vi "Zaber A Series Joystick Configurator.vi"() -> ()   [LabVIEW 2015]
doc: "This VI is a helper for reading and changing the axis and button settings for an X-JOY3 joystick. It can also serve as an example for creating custom joystick initialization routines.\n\n<b>Note this tool only works with Zaber X-series joysticks such as the X-JOY3.</b>"
uses:
  Zaber A Series.lvlib
panel:
  out "Joystick Not \nDetected":bool
  out "Connected":bool
  in  "Joystick Device Number":string="1"
  in  "Disconnect":bool
  in  "VISA resource name":refnum<visa-resource-name>="COM1"
  in  "Connect":bool
  in  "Quit":bool
  in  "Tab Control":enum32{"Axes", "Buttons"}(tab)
  in  "Axis Tab":enum32{"Page 2"}(tab)
  in  "Joystick Axis":u32(ring)=1 items=["Left-Right"=1, "Forward-Back"=2, "Twist"=3]
  in  "Update Axis":bool
  in  "Target Axis Number":i32=1
  in  "Target Device Number":i32=2
  in  "Target Axis Type":u16(ring) items=["Axis", "Lockstep Group", "Virtual Axis"]
  in  "Maximum Speed":i32=100000
  in  "Speed Profile (0: No Change)":u16(ring) items=["No Change", "Linear", "Squared", "Cubed"]
  in  "Axis Direction (0: No Change)":u16(ring) items=["No Change", "Default Direction", "Inverted"]
  in  "Button Tab":enum32{"Page 2"}(tab)
  in  "Update Button":bool
  in  "Joystick Button Number":i32=1 min=1
  in  "Button Event":i32(ring)=1 items=["Pressed"=1, "Released"=2, "Held"=3, "Released After Hold"=4]
  in  "Command List":string[](array[string])
  # "(c) 2017 Zaber Technologies.  ALL RIGHTS RESERVED."
  # "This example allows you to view and edit the configuration of a Zaber ASCII-capable input device such as the X-JOY3.\n\nEnter the serial port and device number of the joystick at upper left and then press the Connect button.\n \nUse the controls in the Axes and Buttons tabs to view and change the settings on the joystick."
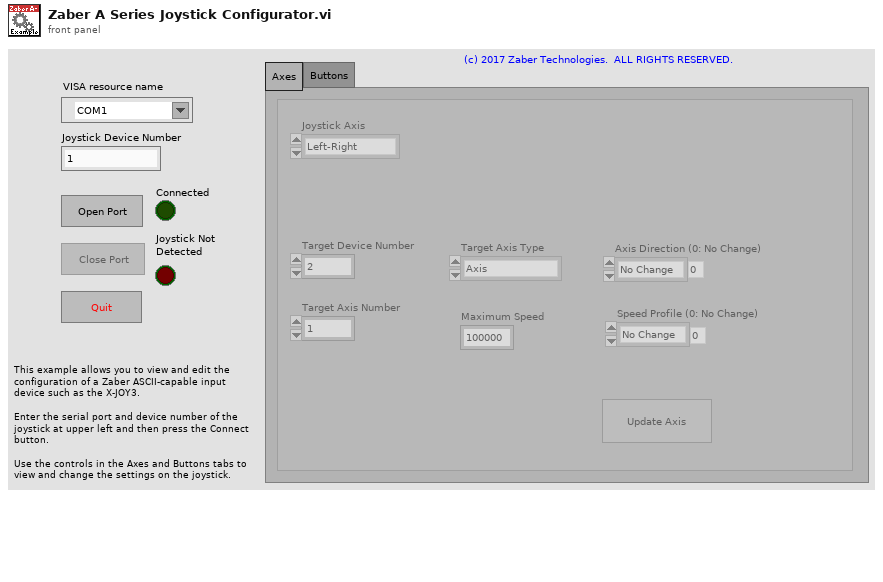
[diagram p1: front panel]
types:
  T1 = enum8{"Enabled", "Disabled", "Disabled and Grayed Out"}
  T2 = cluster{"Device":string, "Axis":string, "Reply Flag":string, "Status":string, "Warning Flags":string, "Data":string}
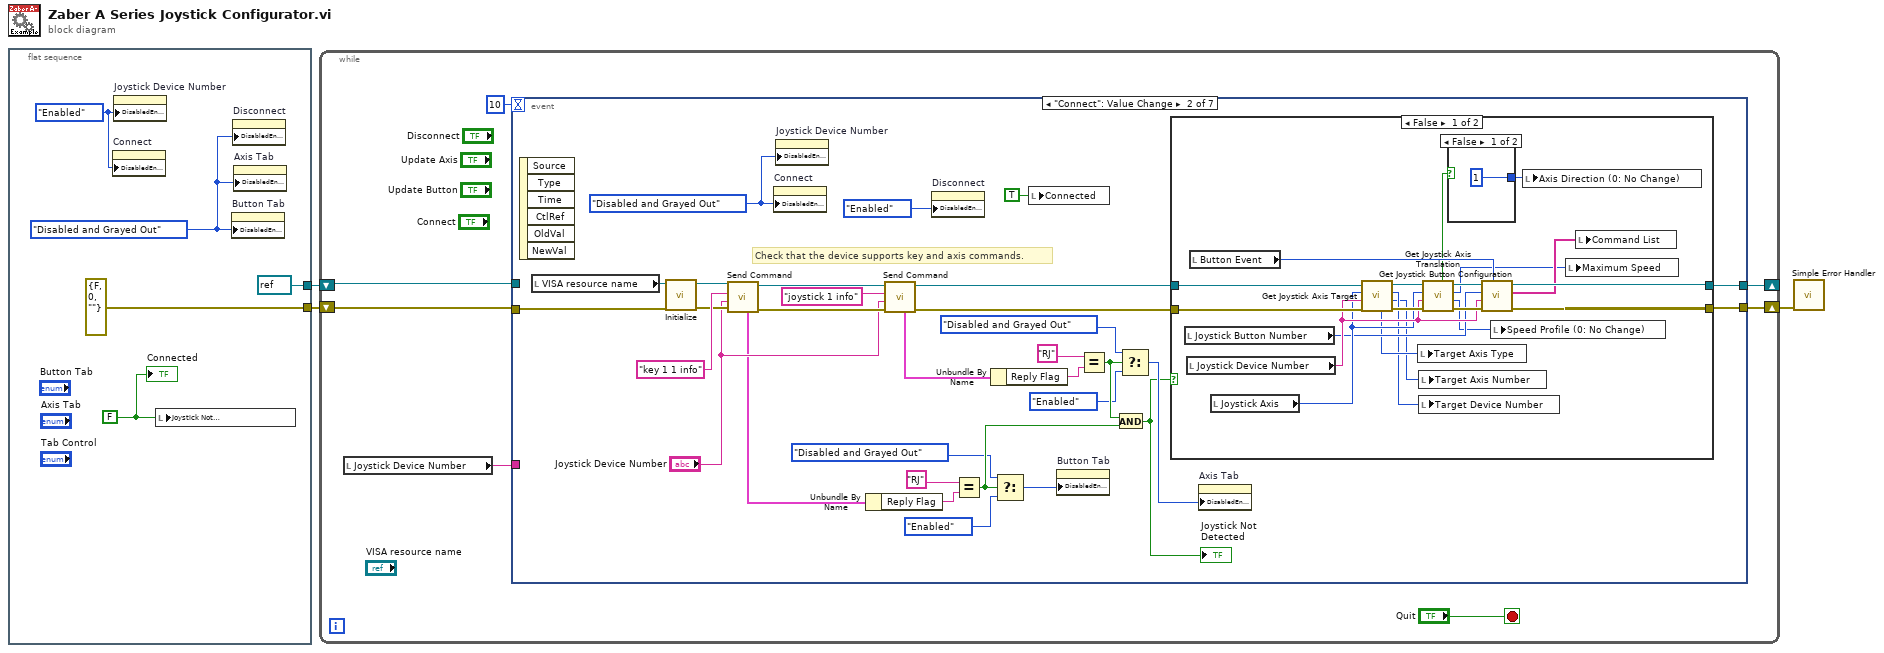
[diagram p0: block diagram]
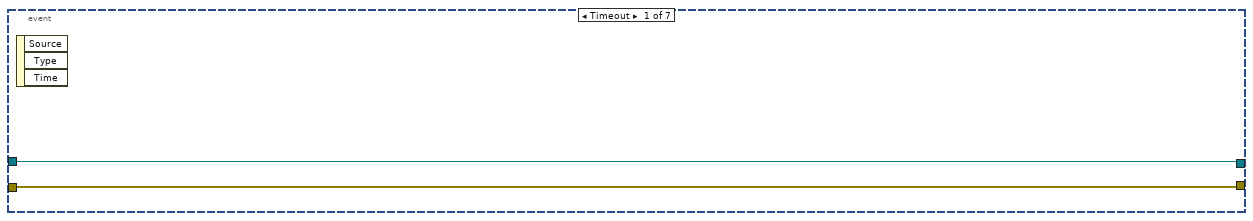
[diagram p2: hidden frame]
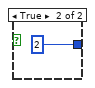
[diagram p3: hidden frame]
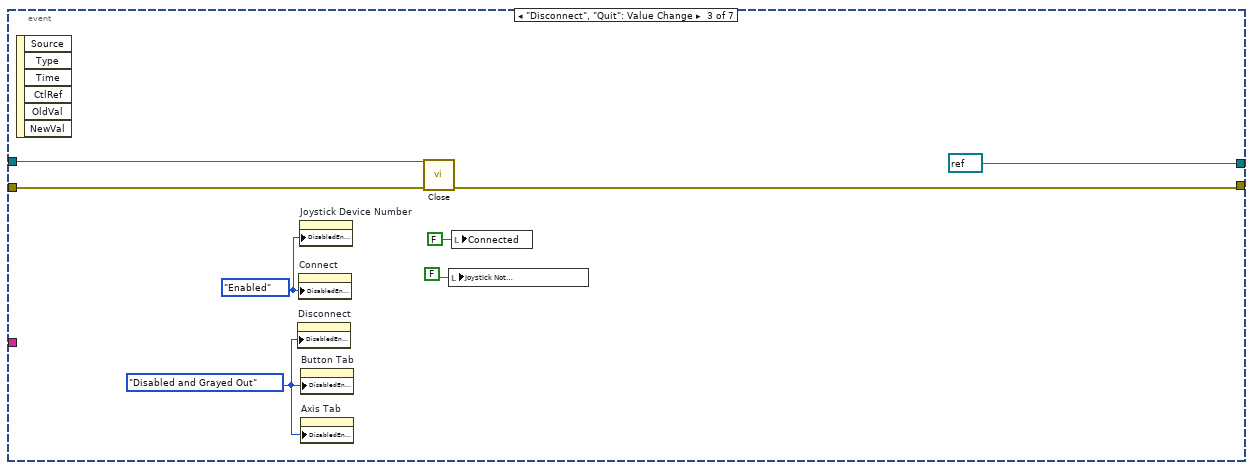
[diagram p5: hidden frame]
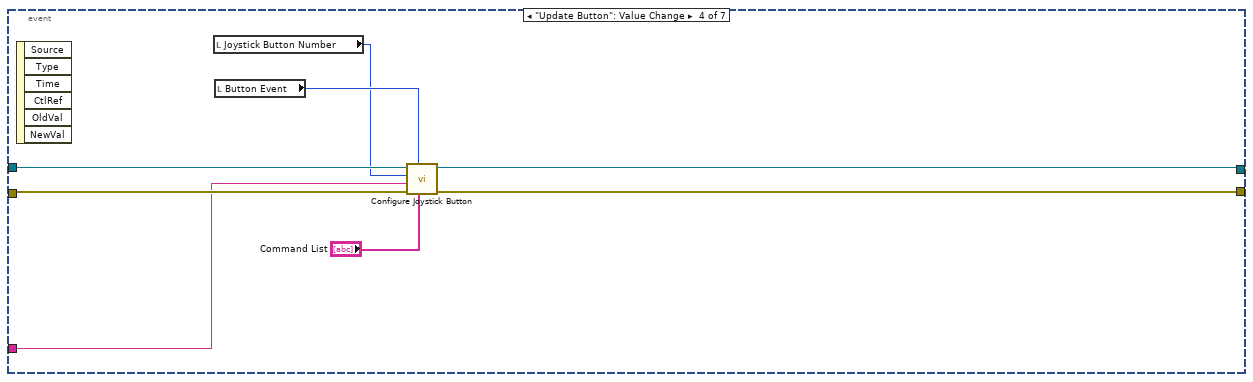
[diagram p6: hidden frame]
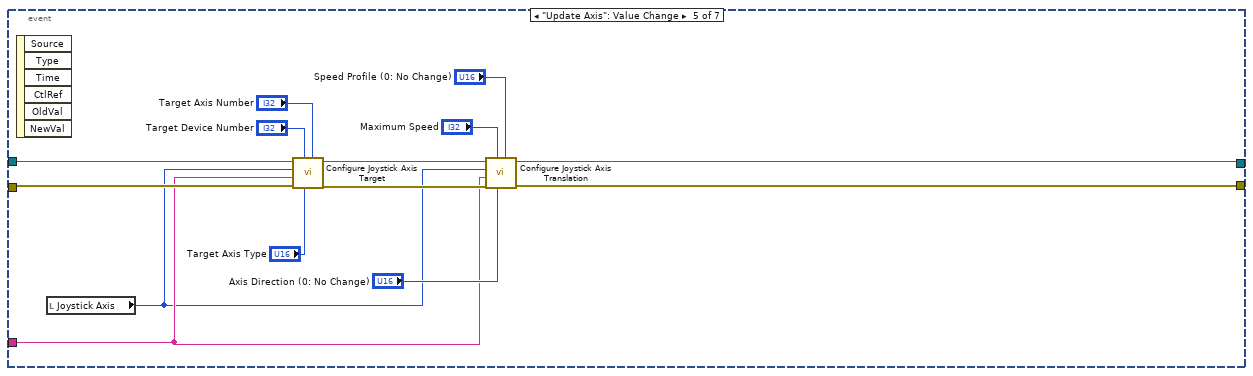
[diagram p7: hidden frame]
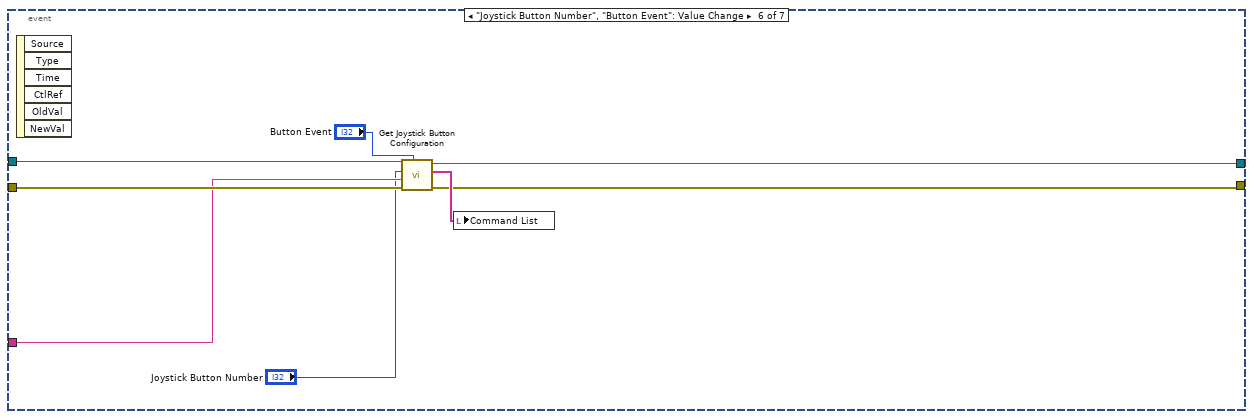
[diagram p8: hidden frame]
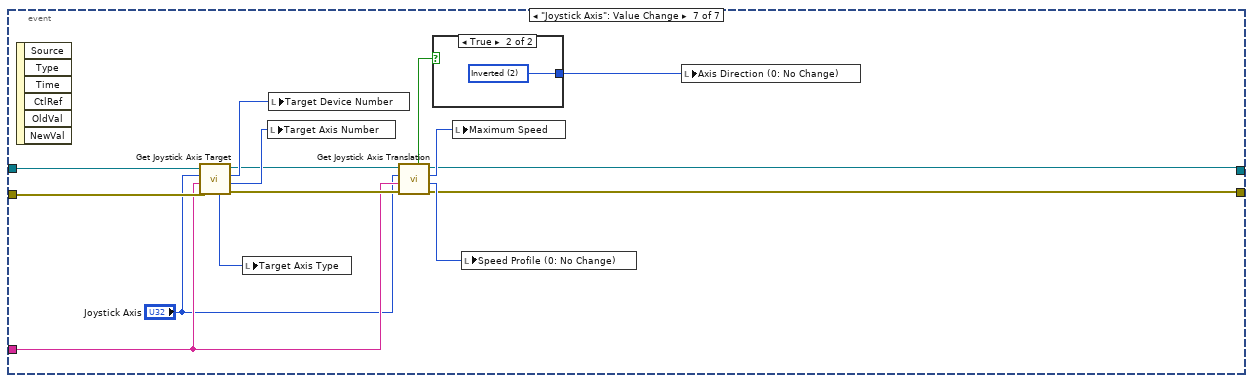
[diagram p9: hidden frame]
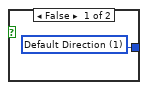
[diagram p10: hidden frame]
diagram:
  n1 = flat-sequence {
    tunnel: [errorcluster {"status"=FALSE, "code"=0, "source"=""} ("error out")] -> w3
    tunnel: [refnum<visa-resource-name> refnum ("VISA resource name out")] -> w1
    frame #0 {
      w5 = T1."Enabled" ("Disabled")
      w7 = T1."Disabled and Grayed Out" ("Disabled")
      w6 = FALSE
      n2 = property on="Connect" class="Bool"("DisabledEnum"=w5) -> ()  [unwired: 2 in, 2 out]
      n3 = property on="Joystick Device Number" class="Str"("DisabledEnum"=w5) -> ()  [unwired: 2 in, 2 out]
      n4 = local write "Joystick Not \nDetected"(w6) -> ()
      n5 = property on="Button Tab" class="TabCtl (strict)"("DisabledEnum"=w7) -> ()  [unwired: 2 in, 2 out]
      n6 = property on="Disconnect" class="Bool"("DisabledEnum"=w7) -> ()  [unwired: 2 in, 2 out]
      n7 = property on="Axis Tab" class="TabCtl (strict)"("DisabledEnum"=w7) -> ()  [unwired: 2 in, 2 out]
      "Connected" <- w6
    }
  }
  n8 = while {
    shift-right: [w12] -> w2
    shift-left: w3 -> [w13]
    shift-right: [w11] -> _
    shift-left: w1 -> [w14]
    stop <- "Quit" stop-if-true
    n9 = local read "Joystick Device Number"() -> (w9:string)
    n10 = event shown="[1] \"Connect\": Value Change" {
      selector: _ -> [_ _ _ _ _ _ _]
      dyn-events: _ -> [_ _ _ _ _ _ _]
      timeout: 10 -> [_ _ _ _ _ _ _]
      tunnel: w14 -> [w17 _ w78 w87 w94 w109 w116]
      tunnel: w13 -> [w16 w28 w77 w85 w93 w107 w115]
      tunnel: [w17 w25 refnum<visa-resource-name> refnum ("VISA resource name out") w86 w92 w108 w114] -> w11
      tunnel: [w16 w23 w75 w84 w91 w106 w113] -> w12
      tunnel: w9 -> [_ _ _ w83 w90 w105 w112]
      event Timeout {
        n11 = event-data() -> ()  [unwired: 1 in, 3 out]
      }
      event "Connect": Value Change {
        w27 = T1."Disabled and Grayed Out" ("Disabled")
        # "Check that the device supports key and axis commands."
        n12 = event-data() -> ()  [unwired: 1 in, 6 out]
        n13 = local read "VISA resource name"() -> (w21:refnum<visa-resource-name>)
        n14 = call "Initialize.vi"("error in (no error)"=w28, "VISA resource name"=w21) -> ("error out"=w32:errorcluster, "VISA resource name out"=w31:refnum<visa-resource-name>)  [unwired: 8 in]
        n15 = call "Send Command.vi"("error in (no error)"=w32, "Device and Axis"="Joystick Device Number", "Command"="key 1 1 info", "VISA resource name"=w31) -> ("error out"=w41:errorcluster, "VISA resource name out"=w40:refnum<visa-resource-name>, "First Response Bundle"=w19:T2)  [unwired: 2 in, 3 out]
        n16 = property on="Connect" class="Bool"("DisabledEnum"=w27) -> ()  [unwired: 2 in, 2 out]
        n17 = property on="Joystick Device Number" class="Str"("DisabledEnum"=w27) -> ()  [unwired: 2 in, 2 out]
        n18 = Unbundle By Name(w19) -> ("Reply Flag"=w35:string)
        n19 = call "Send Command.vi"("error in (no error)"=w41, "Device and Axis"="Joystick Device Number", "Command"="joystick 1 info", "VISA resource name"=w40) -> ("error out"=w24:errorcluster, "VISA resource name out"=w26:refnum<visa-resource-name>, "First Response Bundle"=w18:T2)  [unwired: 2 in, 3 out]
        n20 = property on="Disconnect" class="Bool"("DisabledEnum"=T1."Enabled" ("Disabled")) -> ()  [unwired: 2 in, 2 out]
        n21 = Equal?(x="RJ", y=w35) -> (x = y?=w48:bool)
        n22 = Unbundle By Name(w18) -> ("Reply Flag"=w43:string)
        n23 = Select(t=T1."Disabled and Grayed Out" ("Disabled"), s=w48, f=T1."Enabled" ("Disabled")) -> (s? t:f=w37:T1)
        n24 = local write "Connected"(TRUE ("Connected")) -> ()
        n25 = property on="Button Tab" class="TabCtl (strict)"("DisabledEnum"=w37) -> ()  [unwired: 2 in, 2 out]
        n26 = Equal?(x="RJ", y=w43) -> (x = y?=w47:bool)
        n27 = And(x=w47, y=w48) -> (x .and. y?=w22:bool)
        "Joystick Not \nDetected" <- w22
        n28 = Select(t=T1."Disabled and Grayed Out" ("Disabled"), s=w47, f=T1."Enabled" ("Disabled")) -> (s? t:f=w46:T1)
        n29 = case shown="False" w22 {
          tunnel: w26 -> [w68 w71]
          tunnel: [w65 w71] -> w25
          tunnel: w24 -> [w64 w72]
          tunnel: [w61 w72] -> w23
          frame False {
            n30 = local read "Joystick Button Number"() -> (w58:i32)
            n31 = local read "Joystick Device Number"() -> (w60:string)
            n32 = local read "Button Event"() -> (w57:i32)
            n33 = local read "Joystick Axis"() -> (w59:u32)
            n34 = call "Get Joystick Axis Target.vi"("error in (no error)"=w64, "Joystick Device Number"=w60, "Joystick Axis Number (1)"=w59, "VISA resource name"=w68) -> ("error out"=w63:errorcluster, "Target Axis Number"=w51:i32, "Target Device Number"=w52:i32, "VISA resource name out"=w67:refnum<visa-resource-name>, "Target Axis Type"=w55:u16)  [unwired: 3 in]
            n35 = local write "Target Axis Type"(w55) -> ()
            n36 = local write "Target Axis Number"(w51) -> ()
            n37 = local write "Target Device Number"(w52) -> ()
            n38 = call "Get Joystick Axis Translation.vi"("error in (no error)"=w63, "Joystick Device Number"=w60, "Joystick Axis Number (1)"=w59, "VISA resource name"=w67) -> ("error out"=w62:errorcluster, "Target Speed Profile"=w54:u16, "Maximum Speed"=w53:i32, "VISA resource name out"=w66:refnum<visa-resource-name>, "Joystick Axis Inverted"=w50:bool)  [unwired: 2 in, 1 out]
            n39 = case shown="False" w50 {
              tunnel: [1 2] -> w49
              frame False {
              }
              frame True {
              }
            }
            n40 = call "Get Joystick Button Configuration.vi"("Event Type (1: pressed)"=w57, "error in (no error)"=w62, "Joystick Device Number"=w60, "Key Index (1)"=w58, "VISA resource name"=w66) -> ("error out"=w61:errorcluster, "Command List"=w56:string[], "VISA resource name out"=w65:refnum<visa-resource-name>)  [unwired: 4 in]
            n41 = local write "Speed Profile (0: No Change)"(w54) -> ()
            n42 = local write "Axis Direction (0: No Change)"(w49) -> ()
            n43 = local write "Maximum Speed"(w53) -> ()
            n44 = local write "Command List"(w56) -> ()
          }
          frame True {
          }
        }
        n45 = property on="Axis Tab" class="TabCtl (strict)"("DisabledEnum"=w46) -> ()  [unwired: 2 in, 2 out]
      }
      event "Disconnect", "Quit": Value Change {
        w79 = T1."Disabled and Grayed Out" ("Disabled")
        w73 = T1."Enabled" ("Disabled")
        n46 = event-data() -> ()  [unwired: 1 in, 6 out]
        n47 = property on="Disconnect" class="Bool"("DisabledEnum"=w79) -> ()  [unwired: 2 in, 2 out]
        n48 = property on="Connect" class="Bool"("DisabledEnum"=w73) -> ()  [unwired: 2 in, 2 out]
        n49 = property on="Joystick Device Number" class="Str"("DisabledEnum"=w73) -> ()  [unwired: 2 in, 2 out]
        n50 = property on="Button Tab" class="TabCtl (strict)"("DisabledEnum"=w79) -> ()  [unwired: 2 in, 2 out]
        n51 = property on="Axis Tab" class="TabCtl (strict)"("DisabledEnum"=w79) -> ()  [unwired: 2 in, 2 out]
        n52 = call "Close.vi"("error in (no error)"=w77, "VISA resource name"=w78) -> ("error out"=w75:errorcluster)  [unwired: 9 in]
        n53 = local write "Joystick Not \nDetected"(FALSE ("Device not\nrecognized")) -> ()
        n54 = local write "Connected"(FALSE ("Connected")) -> ()
      }
      event "Update Button": Value Change {
        n55 = event-data() -> ()  [unwired: 1 in, 6 out]
        n56 = local read "Joystick Button Number"() -> (w81:i32)
        n57 = local read "Button Event"() -> (w82:i32)
        n58 = call "Configure Joystick Button.vi"("Command List"="Command List", "Event Type (1: pressed)"=w82, "error in (no error)"=w85, "Joystick Device Number"=w83, "Key Index (1)"=w81, "VISA resource name"=w87) -> ("error out"=w84:errorcluster, "VISA resource name out"=w86:refnum<visa-resource-name>)  [unwired: 4 in]
      }
      event "Update Axis": Value Change {
        n59 = event-data() -> ()  [unwired: 1 in, 6 out]
        n60 = local read "Joystick Axis"() -> (w89:u32)
        n61 = call "Configure Joystick Axis Target.vi"("Target Axis Number (1)"="Target Axis Number", "Target Axis Type (0: axis)"="Target Axis Type", "Target Device Number (1)"="Target Device Number", "error in (no error)"=w93, "Joystick Device Number"=w90, "Joystick Axis Number (1)"=w89, "VISA resource name"=w94) -> ("error out"=w96:errorcluster, "VISA resource name out"=w95:refnum<visa-resource-name>)  [unwired: 3 in]
        n62 = call "Configure Joystick Axis Translation.vi"("Speed Profile (0: no change)"="Speed Profile (0: No Change)", "Axis Direction (0: no change)"="Axis Direction (0: No Change)", "Maximum Speed (0)"="Maximum Speed", "error in (no error)"=w96, "Joystick Device Number"=w90, "Joystick Axis Number (1)"=w89, "VISA resource name"=w95) -> ("error out"=w91:errorcluster, "VISA resource name out"=w92:refnum<visa-resource-name>)  [unwired: 3 in]
      }
      event "Joystick Button Number", "Button Event": Value Change {
        n63 = event-data() -> ()  [unwired: 1 in, 6 out]
        n64 = call "Get Joystick Button Configuration.vi"("Event Type (1: pressed)"="Button Event", "error in (no error)"=w107, "Joystick Device Number"=w105, "Key Index (1)"="Joystick Button Number", "VISA resource name"=w109) -> ("error out"=w106:errorcluster, "Command List"=w110:string[], "VISA resource name out"=w108:refnum<visa-resource-name>)  [unwired: 4 in]
        n65 = local write "Command List"(w110) -> ()
      }
      event "Joystick Axis": Value Change {
        n66 = event-data() -> ()  [unwired: 1 in, 6 out]
        n67 = call "Get Joystick Axis Target.vi"("error in (no error)"=w115, "Joystick Device Number"=w112, "Joystick Axis Number (1)"="Joystick Axis", "VISA resource name"=w116) -> ("error out"=w118:errorcluster, "Target Axis Number"=w120:i32, "Target Device Number"=w119:i32, "VISA resource name out"=w117:refnum<visa-resource-name>, "Target Axis Type"=w121:u16)  [unwired: 3 in]
        n68 = local write "Target Axis Type"(w121) -> ()
        n69 = local write "Target Axis Number"(w120) -> ()
        n70 = local write "Target Device Number"(w119) -> ()
        n71 = call "Get Joystick Axis Translation.vi"("error in (no error)"=w118, "Joystick Device Number"=w112, "Joystick Axis Number (1)"="Joystick Axis", "VISA resource name"=w117) -> ("error out"=w113:errorcluster, "Target Speed Profile"=w123:u16, "Maximum Speed"=w122:i32, "VISA resource name out"=w114:refnum<visa-resource-name>, "Joystick Axis Inverted"=w124:bool)  [unwired: 2 in, 1 out]
        n72 = case shown="True" w124 {
          tunnel: [w126 w127] -> w125
          frame False {
            w126 = u16 1 items=["No Change", "Default Direction", "Inverted"] ("Axis Direction (0: No Change)")
          }
          frame True {
            w127 = u16 2 items=["No Change", "Default Direction", "Inverted"] ("Axis Direction (0: No Change)")
          }
        }
        n73 = local write "Maximum Speed"(w122) -> ()
        n74 = local write "Speed Profile (0: No Change)"(w123) -> ()
        n75 = local write "Axis Direction (0: No Change)"(w125) -> ()
      }
    }
  }
  n76 = call <vilib>:"Simple Error Handler.vi"("error in (no error)"=w2) -> ()  [unwired: 4 in, 5 out]
